vi "Save Event Description.vi"(9 "Event Description":string, 11 "VI in":refnum<class "VI.lvclass">) -> (0 "error out":errorcluster, 3 "VI Out":refnum<class "VI.lvclass">)   [LabVIEW 2019, in "Panther Dashboard.lvlib"]
uses:
  Panther Dashboard.lvlib
  Class/VI/VI.lvclass
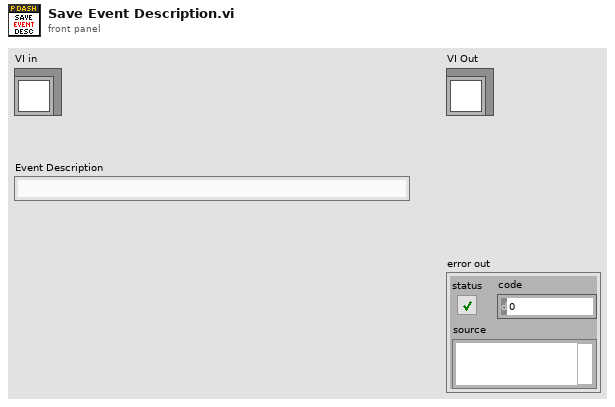
[diagram p1: front panel]
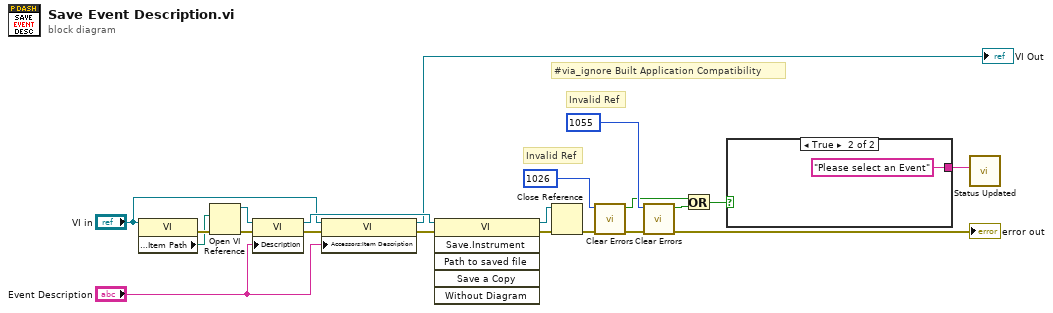
[diagram p0: block diagram]
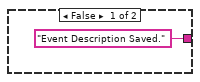
[diagram p2: hidden frame]
diagram:
  # "#via_ignore Built Application Compatibility"
  # "Invalid Ref"
  # "Invalid Ref"
  n1 = property class="VI"(reference="VI in") -> (error out=w18:errorcluster, "Accessors:Item Path"=w5:path)  [unwired: 1 in, 1 out]
  n2 = Open VI Reference(vi path=w5, error in (no error)=w18) -> (vi reference=w4:refnum<vi>, error out=w17:errorcluster)  [unwired: 4 in]
  n3 = property class="VI"(reference=w4, error in=w17, "Description"="Event Description") -> (reference out=w13:refnum<vi>, error out=w15:errorcluster)
  n4 = property class="VI"(reference="VI in", error in=w15, "Accessors:Item Description"="Event Description") -> (reference out=→"VI Out":refnum<class "VI.lvclass">, error out=w14:errorcluster)
  n5 = invoke class="VI" method="Save.Instrument"(reference=w13, error in=w14) -> (reference out=w1:refnum<vi>, error out=w21:errorcluster)  [unwired: 4 in, 4 out]
  n6 = Close Reference(reference=w1, error in (no error)=w21) -> (error out=w16:errorcluster)
  n7 = call <vilib>:"Clear Errors.vi"("error in (no error)"=w16, "specific error code to clear (0: all)"=1026) -> ("error out"=w19:errorcluster, "specific error cleared?"=w8:bool)  [unwired: 4 in]
  n8 = call <vilib>:"Clear Errors.vi"("error in (no error)"=w19, "specific error code to clear (0: all)"=1055) -> ("error out"=→"error out":errorcluster, "specific error cleared?"=w12:bool)  [unwired: 4 in]
  n9 = Or(x=w8, y=w12) -> (x .or. y?=w9:bool)
  n10 = case shown="True" w9 {
    tunnel: ["Event Description Saved." ("Status") "Please select an Event" ("Status")] -> w7
    frame False {
    }
    frame True {
    }
  }
  n11 = call "Status Updated.vi"("Status"=w7) -> ()  [unwired: 10 in, 1 out]
